vi "Close.vi"(8 "error in (no error)":errorcluster, 11 "PythonSession in":refnum<class "PythonSession.lvclass">) -> (0 "error out":errorcluster)   [LabVIEW 2022 SP3, in "PythonWrapper.lvlib" / "PythonSession.lvclass"]
uses:
  PythonSession.lvclass
  PythonSession.lvclass/PythonSession.ctl
  _BankAction.ctl
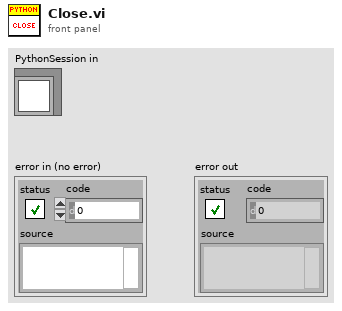
[diagram p1: front panel]
types:
  T1 = typedef "PythonWrapper.lvlib/PythonSession.lvclass/_BankAction.ctl" = enum16{"Get", "Remove"}
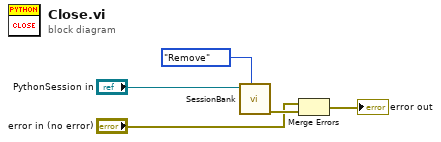
[diagram p0: block diagram]
diagram:
  n1 = call "SessionBank.vi"("Action"=_BankAction."Remove", "PythonSession in"="PythonSession in") -> ("error out"=w3:errorcluster)  [unwired: 8 in, 1 out]
  n2 = Merge Errors("error in (no error)", w3) -> (→"error out":errorcluster)
